vi "Add Parallel Block.vi"(8 "error in (no error)":errorcluster, 11 "AutomationContext in":refnum<class "AutomationContext.lvclass">) -> (0 "error out":errorcluster, 3 "AutomationContext out":refnum<class "AutomationContext.lvclass">)   [LabVIEW 2023, in "Automation.lvlib" / "AutomationContext.lvclass"]
uses:
  AutomationContext.lvclass
  AutomationContext.lvclass/AutomationContext.ctl
  Parallel Block.ctl
  Automation Intent.ctl
  Intent Action.ctl
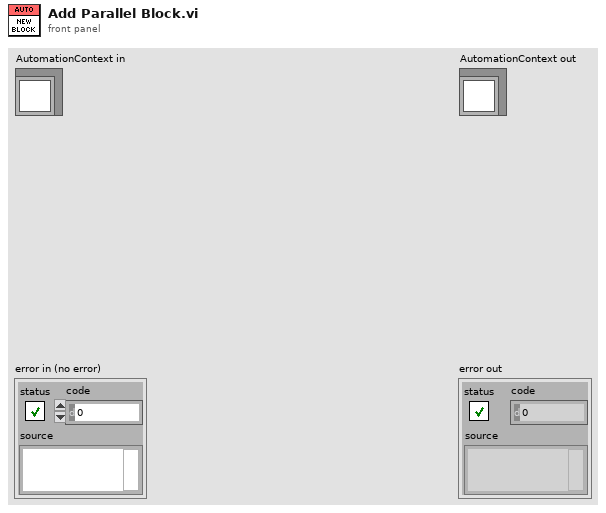
[diagram p1: front panel]
types:
  T1 = typedef "Automation.lvlib/AutomationContext.lvclass/Parallel Block.ctl" = cluster{"Tasks":T2[]}
  T2 = typedef "Automation.lvlib/AutomationContext.lvclass/Automation Intent.ctl" = cluster{"Action":T3, "Parameters":variant, "Correlation ID":u32}
  T3 = typedef "Automation.lvlib/AutomationContext.lvclass/Intent Action.ctl" = enum16{"Next Field", "Next Lane", "Set Power", "Reset Power", "Autofocus", "Start Streaming", "Delay", "Finish Run", "Open Shutter", "Close Shutter"}
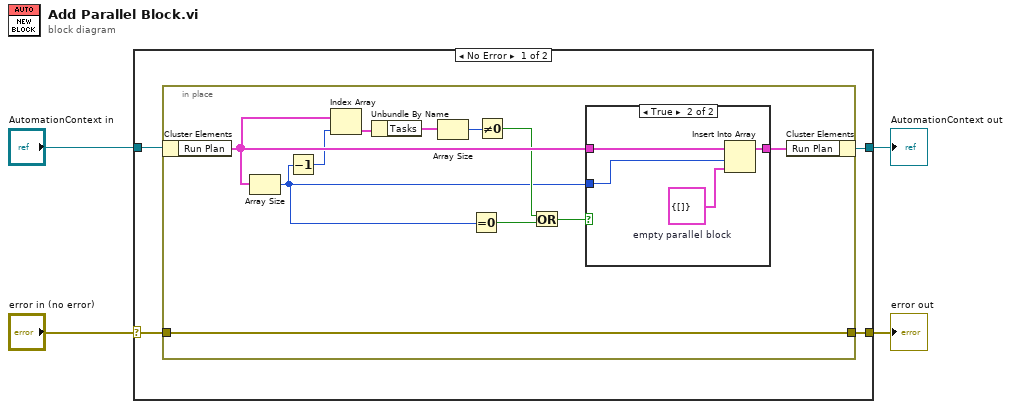
[diagram p0: block diagram]
diagram:
  n1 = case shown="No Error" "error in (no error)" {
    selector: "error in (no error)" -> [w6 w26]
    tunnel: [w5 w26] -> w3
    tunnel: [w7 w25] -> w1
    tunnel: "AutomationContext in" -> [w8 w25]
    frame No Error {
      n2 = in-place {
        in-place-border: w6 -> [w13]
        in-place-border: [w13] -> w5
        n3 = in-place-cluster #1(w8) -> ("Run Plan"=w18:T1[])
        n4 = Array Size(array=w18) -> (size(s)=w11:i32)
        n5 = Decrement(x=w11) -> (x-1=w17:i32)
        n6 = Index Array(array=w18, index=w17) -> (element=w16:T1)
        n7 = Unbundle By Name(w16) -> ("Tasks"=w15:T2[])
        n8 = Array Size(array=w15) -> (size(s)=w14:i32)
        n9 = Equal To 0?(x=w11) -> (x = 0?=w10:bool)
        n10 = Not Equal To 0?(x=w14) -> (x != 0?=w12:bool)
        n11 = Or(x=w12, y=w10) -> (x .or. y?=w9:bool)
        n12 = case shown="True" w9 {
          tunnel: w18 -> [w20 w24]
          tunnel: [w20 w23] -> w19
          tunnel: w11 -> [_ w21]
          frame False {
            # "Don't add successive\nempty parallel blocks"
          }
          frame True {
            w22 = T1 {"Tasks"=[]}  # empty parallel block
            n13 = Insert Into Array(array=w24, index=w21, new element=w22) -> (w23:T1[])
          }
        }
        n14 = in-place-cluster #1("Run Plan"=w19) -> (w7:refnum<class "AutomationContext.lvclass">)
      }
    }
    frame Error {
    }
  }
  "error out" <- w3
  "AutomationContext out" <- w1
